vi "SCCSup Dialog - Compare VIs.vi"(8 "error in (no error)":errorcluster) -> (0 "error out":errorcluster, 2 "cancelled?":bool, 3 "compare options out":T1)   [LabVIEW 2017]
uses:
  <vilib>/SourceControl/sccapi/SCCAPI VI Compare Options.ctl
  <vilib>/SourceControl/sccapi/NI_SCC.lvlib
panel:
  in  "BD pos/size changes":bool caption="BD Position/size changes"
  in  "BD cosmetic changes":bool caption="Cosmetic changes"
  in  "Block Diagram":bool=TRUE
  in  "FP pos/size changes":bool caption="Position/size changes"
  in  "Front Panel":bool=TRUE
  in  "VI properties":bool
  in  "compare":bool
  in  "Cancel":bool
  in  "Help":bool
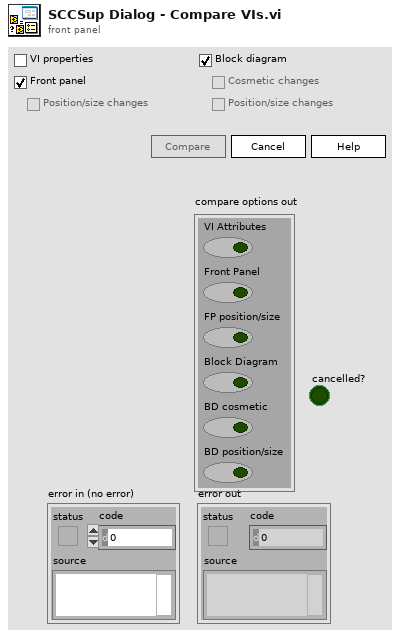
[diagram p1: front panel]
types:
  T1 = typedef "NI_SCC.lvlib/SCCAPI VI Compare Options.ctl" = cluster{"VI Attributes":bool, "Front Panel":bool, "FP position/size":bool, "Block Diagram":bool, "BD cosmetic":bool, "BD position/size":bool}
  T2 = cluster{"Boolean array[0]":bool, "Boolean array[1]":bool, "Boolean array[2]":bool, "Boolean array[3]":bool, "Boolean array[4]":bool, "Boolean array[5]":bool}
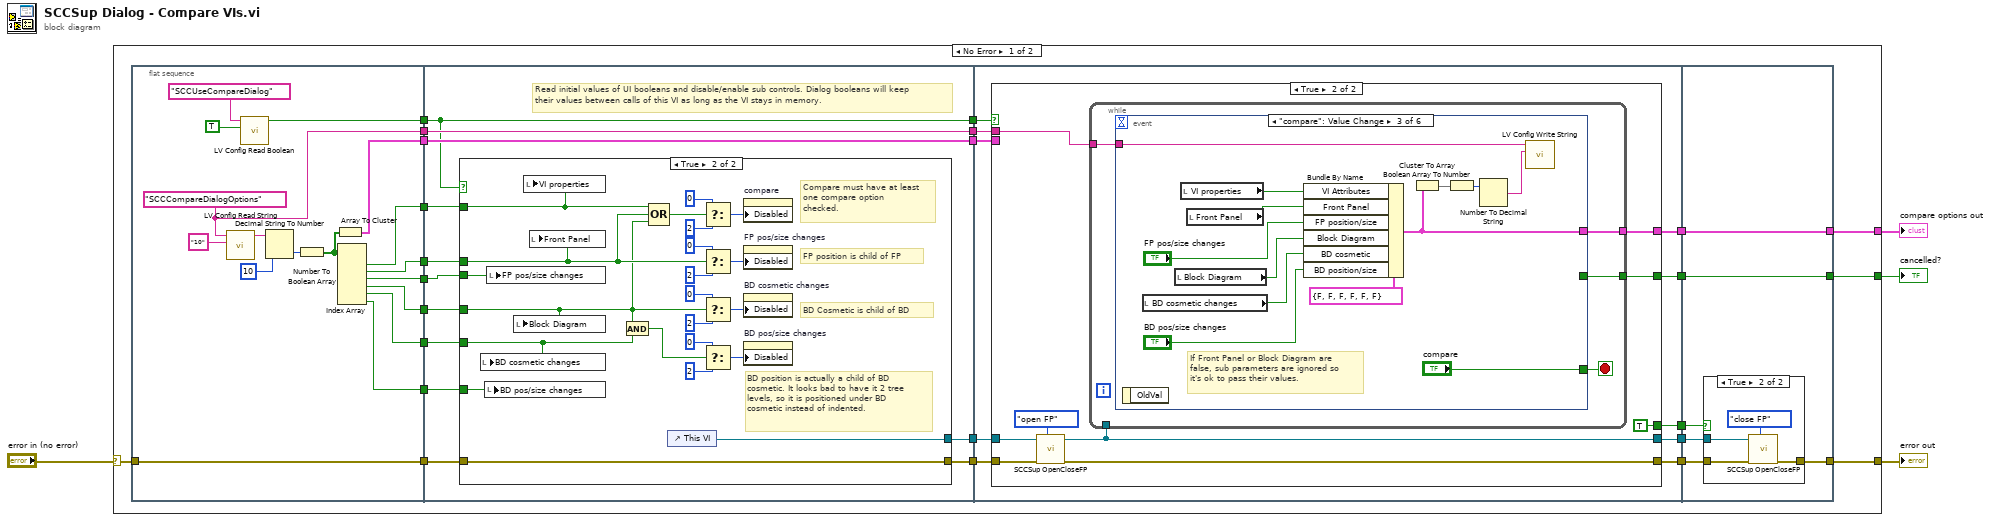
[diagram p0: block diagram]
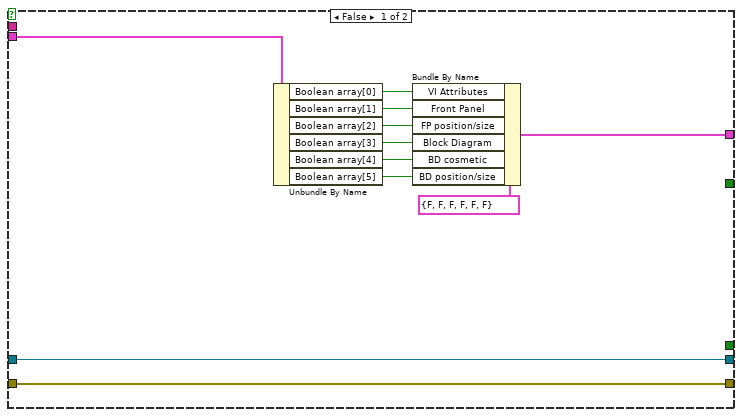
[diagram p3: hidden frame]
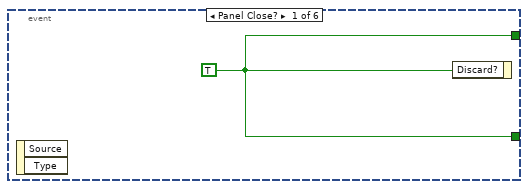
[diagram p4: hidden frame]
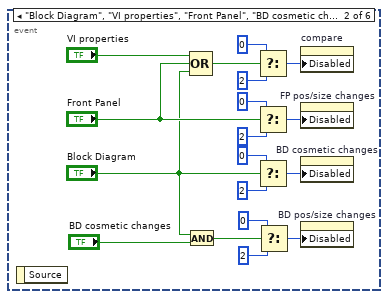
[diagram p5: hidden frame]
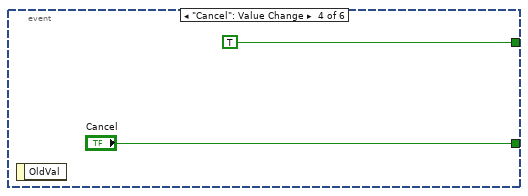
[diagram p6: hidden frame]
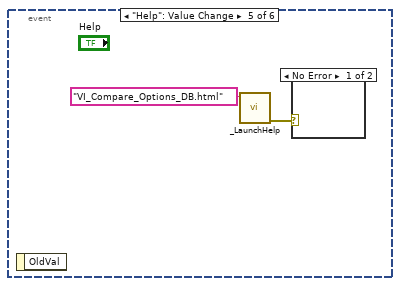
[diagram p7: hidden frame]
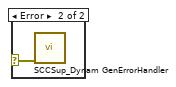
[diagram p8: hidden frame]
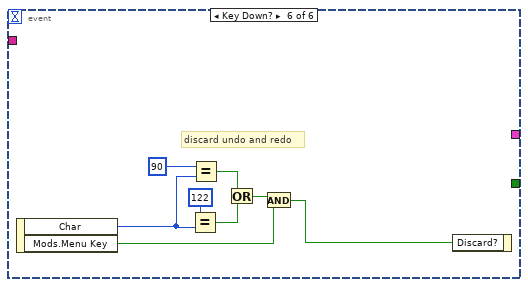
[diagram p9: hidden frame]
diagram:
  n1 = case shown="No Error" "error in (no error)" {
    selector: "error in (no error)" -> [w26 w171]
    tunnel: [w23 w171] -> w3
    tunnel: [w21 _] -> w2
    tunnel: [w19 _] -> w1
    frame No Error {
      n2 = flat-sequence {
        tunnel: w26 -> [w45]
        tunnel: [w45] -> w18
        tunnel: [w38] -> w17
        tunnel: [w37] -> w16
        tunnel: [w36] -> w15
        tunnel: [w35] -> w14
        tunnel: [w34] -> w13
        tunnel: [w33] -> w12
        tunnel: [w32] -> w10
        tunnel: [w31] -> w9
        tunnel: [w29] -> w6
        tunnel: [w57] -> w28
        tunnel: [w46] -> w25
        tunnel: w18 -> [w47]
        tunnel: w17 -> [w56]
        tunnel: w16 -> [w55]
        tunnel: w15 -> [w54]
        tunnel: w14 -> [w53]
        tunnel: w13 -> [w52]
        tunnel: w12 -> [w51]
        tunnel: [w48] -> w11
        tunnel: w10 -> [w48]
        tunnel: w9 -> [w50]
        tunnel: [w50] -> w8
        tunnel: [w49] -> w7
        tunnel: w6 -> [w49]
        tunnel: [w89] -> w27
        tunnel: w28 -> [w90]
        tunnel: w25 -> [w88]
        tunnel: [w87] -> w24
        tunnel: [w86] -> w22
        tunnel: [w85] -> w20
        tunnel: w11 -> [w83]
        tunnel: w8 -> [w82]
        tunnel: w7 -> [w84]
        tunnel: [w81] -> w5
        tunnel: w27 -> [w165]
        tunnel: w24 -> [w164]
        tunnel: [w163] -> w23
        tunnel: w22 -> [w162]
        tunnel: [w162] -> w21
        tunnel: w20 -> [w161]
        tunnel: [w161] -> w19
        tunnel: w5 -> [w160]
        frame #0 {
          w31 = "SCCCompareDialogOptions" ("key")
          n3 = call <resource>:"LV Config Read String.vi"("default value"="10", "key"=w31) -> ("value"=w39:string)  [unwired: 3 in, 2 out]
          n4 = call <resource>:"LV Config Read Boolean.vi"("default value"=TRUE, "key"="SCCUseCompareDialog") -> ("value"=w32:bool)  [unwired: 3 in, 2 out]
          n5 = Decimal String To Number(string=w39, default (0L)=10 ("default (0 I32)")) -> (number=w42:i32)  [unwired: 1 in, 1 out]
          n6 = Number To Boolean Array(number=w42) -> (Boolean array=w30:bool[])
          n7 = Array To Cluster(array=w30) -> (cluster=w29:T2)
          n8 = Index Array(array=w30) -> (element #1=w38:bool, element #2=w37:bool, element #3=w36:bool, element #4=w35:bool, element #5=w34:bool, element #6=w33:bool)  [unwired: 6 in]
        }
        frame #1 {
          # "Read initial values of UI booleans and disable/enable sub controls. Dialog booleans will keep their values between calls of this VI as long as the VI stays in memory."
          n9 = case shown="True" w48 {
            tunnel: [_ w70] -> w57
            tunnel: w56 -> [_ w65]
            tunnel: w55 -> [_ w64]
            tunnel: w54 -> [_ w63]
            tunnel: w53 -> [_ w62]
            tunnel: w52 -> [_ w61]
            tunnel: w51 -> [_ w60]
            tunnel: w47 -> [w58 w59]
            tunnel: [w58 w59] -> w46
            frame False {
            }
            frame True {
              # "BD position is actually a child of BD cosmetic. It looks bad to have it 2 tree levels, so it is positioned under BD cosmetic instead of indented."
              # "BD Cosmetic is child of BD"
              # "FP position is child of FP"
              # "Compare must have at least one compare option checked."
              n10 = local write "BD cosmetic changes"(w61) -> ()
              n11 = local write "BD pos/size changes"(w60) -> ()
              n12 = local write "FP pos/size changes"(w63) -> ()
              n13 = local write "Block Diagram"(w62) -> ()
              n14 = local write "VI properties"(w65) -> ()
              n15 = local write "Front Panel"(w64) -> ()
              n16 = And(x=w62, y=w61) -> (x .and. y?=w66:bool)
              n17 = Compound Arithmetic op=OR(w65, w64, w62) -> (w73:bool)
              n18 = control-ref of="This VI"() -> (w70:refnum<vi>)
              n19 = Select(t=u8 0 ("Disabled"), s=w73, f=u8 2 ("Disabled")) -> (s? t:f=w74:u8)
              n20 = Select(t=u8 0 ("Disabled"), s=w64, f=u8 2 ("Disabled")) -> (s? t:f=w79:u8)
              n21 = Select(t=u8 0 ("Disabled"), s=w62, f=u8 2 ("Disabled")) -> (s? t:f=w80:u8)
              n22 = Select(t=u8 0 ("Disabled"), s=w66, f=u8 2 ("Disabled")) -> (s? t:f=w67:u8)
              n23 = property on="compare" class="Bool"("Disabled"=w74) -> ()  [unwired: 2 in, 2 out]
              n24 = property on="FP pos/size changes" class="Bool (strict)"("Disabled"=w79) -> ()  [unwired: 2 in, 2 out]
              n25 = property on="BD cosmetic changes" class="Bool (strict)"("Disabled"=w80) -> ()  [unwired: 2 in, 2 out]
              n26 = property on="BD pos/size changes" class="Bool (strict)"("Disabled"=w67) -> ()  [unwired: 2 in, 2 out]
            }
          }
        }
        frame #2 {
          n27 = case shown="True" w83 {
            tunnel: w90 -> [w100 w109]
            tunnel: [w100 w108] -> w89
            tunnel: w88 -> [w101 w107]
            tunnel: [w101 w106] -> w87
            tunnel: [_ w105] -> w86
            tunnel: [w99 w104] -> w85
            tunnel: w84 -> [w97 _]
            tunnel: w82 -> [_ w103]
            tunnel: [_ TRUE] -> w81
            frame False {
              n28 = Unbundle By Name(w97) -> ("Boolean array[0]"=w96:bool, "Boolean array[1]"=w95:bool, "Boolean array[2]"=w94:bool, "Boolean array[3]"=w93:bool, "Boolean array[4]"=w92:bool, "Boolean array[5]"=w91:bool)
              n29 = Bundle By Name(cluster=T1 {"VI Attributes"=FALSE, "Front Panel"=FALSE, "FP position/size"=FALSE, "Block Diagram"=FALSE, "BD cosmetic"=FALSE, "BD position/size"=FALSE} ("compare options"), "VI Attributes"=w96, "Front Panel"=w95, "FP position/size"=w94, "Block Diagram"=w93, "BD cosmetic"=w92, "BD position/size"=w91) -> (w99:T1)
            }
            frame True {
              n30 = call <vilib>:"SCCSup OpenCloseFP.vi"("function"=enum16{"open FP", "close FP"}."open FP", "error in (no error)"=w107, "VI Refnum in"=w109) -> ("error out"=w106:errorcluster, "VI Refnum out"=w108:refnum<vi>)  [unwired: 7 in]
              n31 = while {
                tunnel: [w113] -> w105
                tunnel: w108 -> [_]
                tunnel: [w112] -> w104
                tunnel: w103 -> [w111]
                stop <- w114 stop-if-true
                n32 = event shown="[2] \"compare\": Value Change" {
                  selector: _ -> [_ _ _ _ _ _]
                  dyn-events: _ -> [_ _ _ _ _ _]
                  timeout: _ -> [_ _ _ _ _ _]
                  tunnel: [w115 _ "compare" "Cancel" _ _] -> w114
                  tunnel: [w115 _ _ TRUE _ _] -> w113
                  tunnel: [_ _ w138 _ _ _] -> w112
                  tunnel: w111 -> [_ _ w135 _ _ _]
                  event Panel Close? {
                    w115 = TRUE
                    n33 = event-data() -> ()  [unwired: 1 in, 2 out]
                    n34 = event-data("Discard?"=w115) -> ()  [unwired: 1 in, 1 out]
                  }
                  event "Block Diagram", "VI properties", "Front Panel", "BD cosmetic changes": Value Change {
                    n35 = event-data() -> ()  [unwired: 1 in, 1 out]
                    n36 = And(x="Block Diagram", y="BD cosmetic changes") -> (x .and. y?=w117:bool)
                    n37 = Compound Arithmetic op=OR("VI properties", "Front Panel", "Block Diagram") -> (w130:bool)
                    n38 = Select(t=u8 0 ("Disabled"), s=w130, f=u8 2 ("Disabled")) -> (s? t:f=w129:u8)
                    n39 = Select(t=u8 0 ("Disabled"), s="Front Panel", f=u8 2 ("Disabled")) -> (s? t:f=w124:u8)
                    n40 = Select(t=u8 0 ("Disabled"), s="Block Diagram", f=u8 2 ("Disabled")) -> (s? t:f=w123:u8)
                    n41 = Select(t=u8 0 ("Disabled"), s=w117, f=u8 2 ("Disabled")) -> (s? t:f=w119:u8)
                    n42 = property on="compare" class="Bool"("Disabled"=w129) -> ()  [unwired: 2 in, 2 out]
                    n43 = property on="FP pos/size changes" class="Bool (strict)"("Disabled"=w124) -> ()  [unwired: 2 in, 2 out]
                    n44 = property on="BD cosmetic changes" class="Bool (strict)"("Disabled"=w123) -> ()  [unwired: 2 in, 2 out]
                    n45 = property on="BD pos/size changes" class="Bool (strict)"("Disabled"=w119) -> ()  [unwired: 2 in, 2 out]
                  }
                  event "compare": Value Change {
                    # "If Front Panel or Block Diagram are false, sub parameters are ignored so it's ok to pass their values."
                    n46 = event-data() -> ()  [unwired: 1 in, 1 out]
                    n47 = local read "BD cosmetic changes"() -> (w140:bool)
                    n48 = local read "Block Diagram"() -> (w143:bool)
                    n49 = local read "VI properties"() -> (w145:bool)
                    n50 = local read "Front Panel"() -> (w144:bool)
                    n51 = Bundle By Name(cluster=T1 {"VI Attributes"=FALSE, "Front Panel"=FALSE, "FP position/size"=FALSE, "Block Diagram"=FALSE, "BD cosmetic"=FALSE, "BD position/size"=FALSE} ("compare options"), "VI Attributes"=w145, "Front Panel"=w144, "FP position/size"="FP pos/size changes", "Block Diagram"=w143, "BD cosmetic"=w140, "BD position/size"="BD pos/size changes") -> (w138:T1)
                    n52 = Cluster To Array(cluster=w138) -> (array=w134:bool[])
                    n53 = Boolean Array To Number(Boolean array=w134) -> (number=w137:u32)
                    n54 = Number To Decimal String(number=w137) -> (decimal integer string=w136:string)  [unwired: 1 in]
                    n55 = call <resource>:"LV Config Write String.vi"("value"=w136, "key"=w135) -> ()  [unwired: 5 in, 1 out]
                  }
                  event "Cancel": Value Change {
                    n56 = event-data() -> ()  [unwired: 1 in, 1 out]
                  }
                  event "Help": Value Change {
                    n57 = event-data() -> ()  [unwired: 1 in, 1 out]
                    n58 = call <helpdir>:"_LaunchHelp.vi"("HTML filename"="VI_Compare_Options_DB.html" ("Help topic")) -> ("error out"=w150:errorcluster)  [unwired: 6 in]
                    n59 = case shown="No Error" w150 {
                      selector: w150 -> [_ w151]
                      frame No Error {
                      }
                      frame Error {
                        n60 = call <vilib>:"SCCSup_Dynam GenErrorHandler.vi"("error in (no error)"=w151) -> ()  [unwired: 9 in, 2 out]
                      }
                    }
                  }
                  event Key Down? {
                    # "discard undo and redo"
                    n61 = event-data() -> ("Char"=w159:i16, "Mods.Menu Key"=w158:bool)  [unwired: 1 in]
                    n62 = Equal?(x=i16 122, y=w159) -> (x = y?=w154:bool)
                    n63 = Equal?(x=i16 90, y=w159) -> (x = y?=w153:bool)
                    n64 = Or(x=w153, y=w154) -> (x .or. y?=w152:bool)
                    n65 = And(x=w152, y=w158) -> (x .and. y?=w157:bool)
                    n66 = event-data("Discard?"=w157) -> ()  [unwired: 1 in, 1 out]
                  }
                }
              }
            }
          }
        }
        frame #3 {
          n67 = case shown="True" w160 {
            tunnel: w165 -> [_ w169]
            tunnel: w164 -> [w166 w168]
            tunnel: [w166 w167] -> w163
            frame False {
            }
            frame True {
              n68 = call <vilib>:"SCCSup OpenCloseFP.vi"("function"=enum16{"open FP", "close FP"}."close FP", "error in (no error)"=w168, "VI Refnum in"=w169) -> ("error out"=w167:errorcluster)  [unwired: 7 in, 1 out]
            }
          }
        }
      }
    }
    frame Error {
    }
  }
  "error out" <- w3
  "cancelled?" <- w2
  "compare options out" <- w1
